vi "OWIS_SetLimits.vi"(8 "error in (no error)":errorcluster, 10 "Axis":T1=1 items=["1"=1, "2"=2, "3"=3, "4"=4], 11 "DLOwis in":refnum<class "DLOwis.lvclass">) -> (0 "error out":errorcluster, 3 "DLOwis out":refnum<class "DLOwis.lvclass">)   [LabVIEW 2019, in "DLOwis.lvclass"]
uses:
  DLOwis.lvclass
  C:/Dev/TRANCON/Classes/Delay Line/DelayLine.lvclass
  C:/Dev/TRANCON/Classes/GeneralFunctionality/GeneralFunctionality.lvclass
  DelayLineLS4/LS4 axis.ctl
  DelayLineLS4/LS4_parameters.ctl
  GeneralFunctionality/GeneralFunctionality.lvclass/GeneralFunctionality.ctl
  Config/Config.lvclass
  DelayLine.lvclass
  GeneralFunctionality/GeneralFunctionality.lvclass
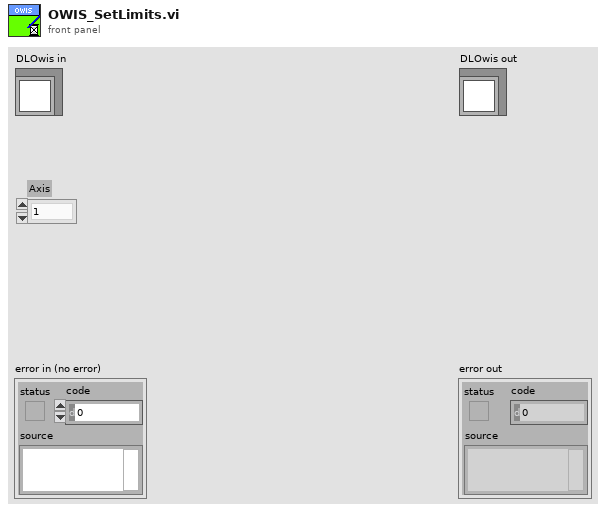
[diagram p1: front panel]
types:
  T1 = typedef "DelayLine.lvclass/LS4 axis.ctl" = u16
  T2 = typedef "DelayLine.lvclass/LS4_parameters.ctl" = string
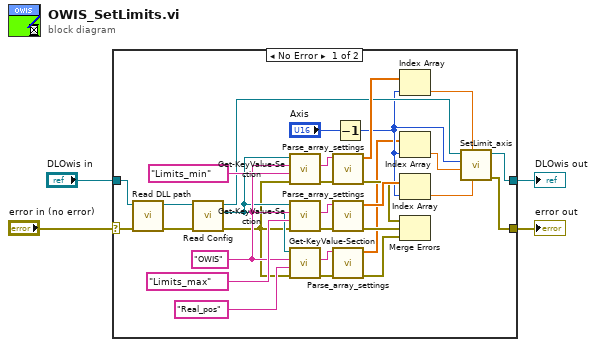
[diagram p0: block diagram]
diagram:
  n1 = case shown="No Error" "error in (no error)" {
    selector: "error in (no error)" -> [w33 w35]
    tunnel: [w19 w36] -> w2
    tunnel: "DLOwis in" -> [w34 w36]
    tunnel: [w18 w35] -> w1
    frame No Error {
      w14 = "OWIS" ("Section")
      n2 = call "Read DLL path.vi"("error in (no error)"=w33, "DelayLine in"=w34) -> ("error out"=w29:errorcluster, "DelayLine out"=w21:refnum<class "DLOwis.lvclass">)  [unwired: 7 in, 1 out]
      n3 = call "Read Config.vi"("error in (no error)"=w29, "GeneralFunctionality en entrée"=w21) -> ("error out"=w12:errorcluster, "Config.lvclass"=w13:refnum<class "Config.lvclass">, "GeneralFunctionality en sortie"=w20:refnum<class "DLOwis.lvclass">)  [unwired: 7 in]
      n4 = call-dynamic "Get-KeyValue-Section.vi"("error in (no error)"=w12, "Key"=T2 "Limits_min" ("Section"), "Section"=w14, "Config in"=w13) -> ("error out"=w31:errorcluster, "Value"=w32:string)  [unwired: 5 in, 1 out]
      n5 = call-dynamic "Get-KeyValue-Section.vi"("error in (no error)"=w12, "Key"=T2 "Limits_max" ("Section"), "Section"=w14, "Config in"=w13) -> ("error out"=w27:errorcluster, "Value"=w26:string)  [unwired: 5 in, 1 out]
      n6 = call-dynamic "Get-KeyValue-Section.vi"("error in (no error)"=w12, "Key"="Real_pos", "Section"=w14, "Config in"=w13) -> ("error out"=w8:errorcluster, "Value"=w9:string)  [unwired: 5 in, 1 out]
      n7 = call "Parse_array_settings.vi"("error in (no error)"=w31, "Value"=w32) -> ("error out"=w23:errorcluster, "Array"=w28:sgl[])  [unwired: 8 in]
      n8 = call "Parse_array_settings.vi"("error in (no error)"=w27, "Value"=w26) -> ("error out"=w22:errorcluster, "Array"=w24:sgl[])  [unwired: 8 in]
      n9 = call "Parse_array_settings.vi"("error in (no error)"=w8, "Value"=w9) -> ("error out"=w7:errorcluster, "Array"=w10:sgl[])  [unwired: 8 in]
      n10 = Decrement(x="Axis") -> (x-1=w11:T1)
      n11 = Index Array(array=w28, index=w11) -> (element=w17:sgl)
      n12 = Index Array(array=w10, index=w11) -> (element=w6:sgl)
      n13 = Index Array(array=w24, index=w11) -> (element=w16:sgl)
      n14 = Merge Errors(w23, w22, w7) -> ()  [unwired: 1 out]
      n15 = call-dynamic "SetLimit_axis.vi"("max"=w16, "min"=w17, "real pos zero"=w6, "Axis"=w11, "DelayLine in"=w20) -> ("error out"=w18:errorcluster, "DelayLine out"=w19:refnum<class "DLOwis.lvclass">)  [unwired: 5 in]
    }
    frame Error {
    }
  }
  "error out" <- w1
  "DLOwis out" <- w2
